vi "Write Record Data.vi"(8 "Error In (no error)":errorcluster, 10 "Record":variant, 11 "Expenses Tracker Balance In":refnum<class "Expenses Tracker Balance.lvclass">) -> (0 "Error Out":errorcluster, 3 "Expenses Tracker Balance Out":refnum<class "Expenses Tracker Balance.lvclass">)   [LabVIEW 2023, in "Expenses Tracker Balance.lvclass"]
uses:
  Expenses Tracker Balance.lvclass
  Expenses Tracker Balance.lvclass/Expenses Tracker Balance.ctl
  Expenses Tracker Record/Public/Ctrls/Balance.ctl
  Expenses Tracker Record/Expenses Tracker Record.lvclass
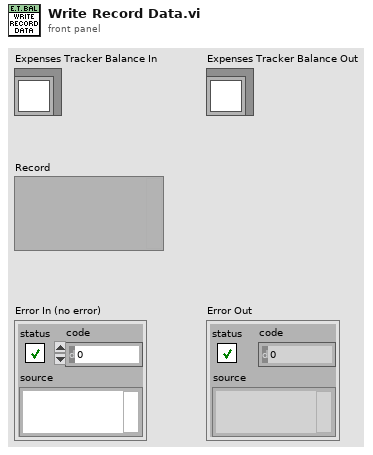
[diagram p1: front panel]
types:
  T1 = typedef "Expenses Tracker Record.lvclass/Balance.ctl" = cluster{"ID":u8, "Value":dbl, "Last_update":timestamp}
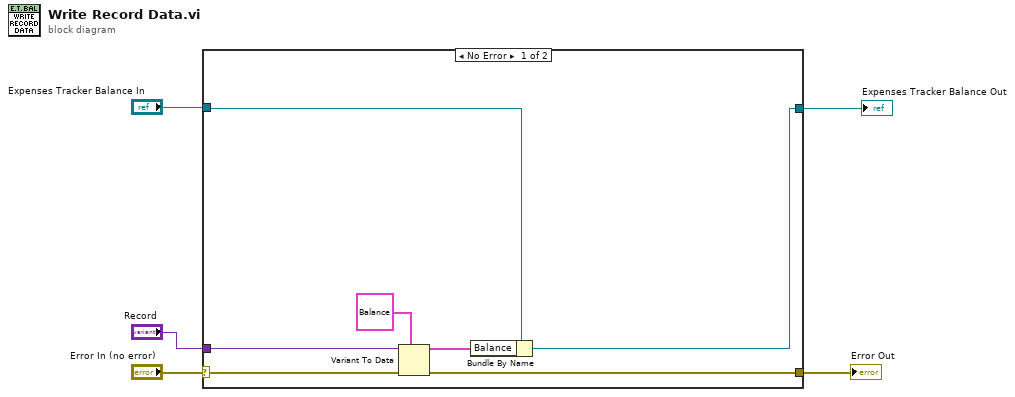
[diagram p0: block diagram]
diagram:
  n1 = case shown="No Error" "Error In (no error)" {
    selector: "Error In (no error)" -> [w10 w14]
    tunnel: [w8 w14] -> w4
    tunnel: [w6 w13] -> w3
    tunnel: "Expenses Tracker Balance In" -> [w7 w13]
    tunnel: "Record" -> [w12 _]
    frame No Error {
      n2 = Variant To Data(error in=w10, type=T1 {"ID"=0, "Value"=0.0, "Last_update"=timestamp(0 s since 1904-01-01)} ("Balance"), Variant=w12) -> (data=w11:T1, error out=w8:errorcluster)
      n3 = Bundle By Name(cluster=w7, "Balance"=w11) -> (w6:refnum<class "Expenses Tracker Balance.lvclass">)
    }
    frame Error {
    }
  }
  "Error Out" <- w4
  "Expenses Tracker Balance Out" <- w3
